vi "LoadController.vi"(8 "error in (no error)":errorcluster, 10 "Actor In":refnum<class "Actor.lvclass">, 11 "Microscope in":refnum<class "Microscope.lvclass">) -> (0 "error out":errorcluster, 3 "Microscope out":refnum<class "Microscope.lvclass">)   [LabVIEW 2020, in "Microscope.lvlib" / "Microscope.lvclass"]
uses:
  Microscope.lvclass
  <vilib>/ActorFramework/Actor/Actor.lvclass
  Component/Device/Device/DataExchange.ctl
  ViewController/Microscope Controller/MicroscopeController.lvclass
  C:/Program Files/National Instruments/LabVIEW 2020/vi.lib/ActorFramework/Actor/Actor.lvclass
  Microscope.lvclass/Microscope.ctl
  Interface/DataListener Messages/OnDataChange Msg/OnDataChange Msg.lvclass/OnDataChange Msg.ctl
  <vilib>/ActorFramework/Message Enqueuer/Message Enqueuer.lvclass/Message Enqueuer.ctl
  <vilib>/ActorFramework/Message Enqueuer/Enqueue.vi
  Interface/DataListener Messages/OnDataChange Msg/OnDataChange Msg.lvclass
  C:/Program Files/National Instruments/LabVIEW 2020/vi.lib/ActorFramework/Message/Message.lvclass
  <vilib>/ActorFramework/Message Priority Queue/Priority Enqueue.vi
  Component/Device/Device/Device.lvclass
  Interface/DataListener/DataListener.lvclass
panel:
  in  "cluster":T1
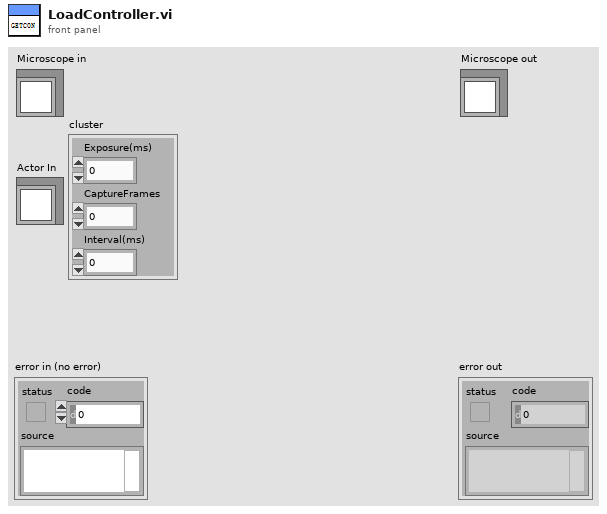
[diagram p1: front panel]
types:
  T1 = cluster{"Exposure(ms)":dbl, "CaptureFrames":dbl, "Interval(ms)":dbl}
  T2 = typedef "DataListener.lvclass/DataExchange.ctl" = cluster{"Source":string, "Destination":string, "Description":string, "value":variant}
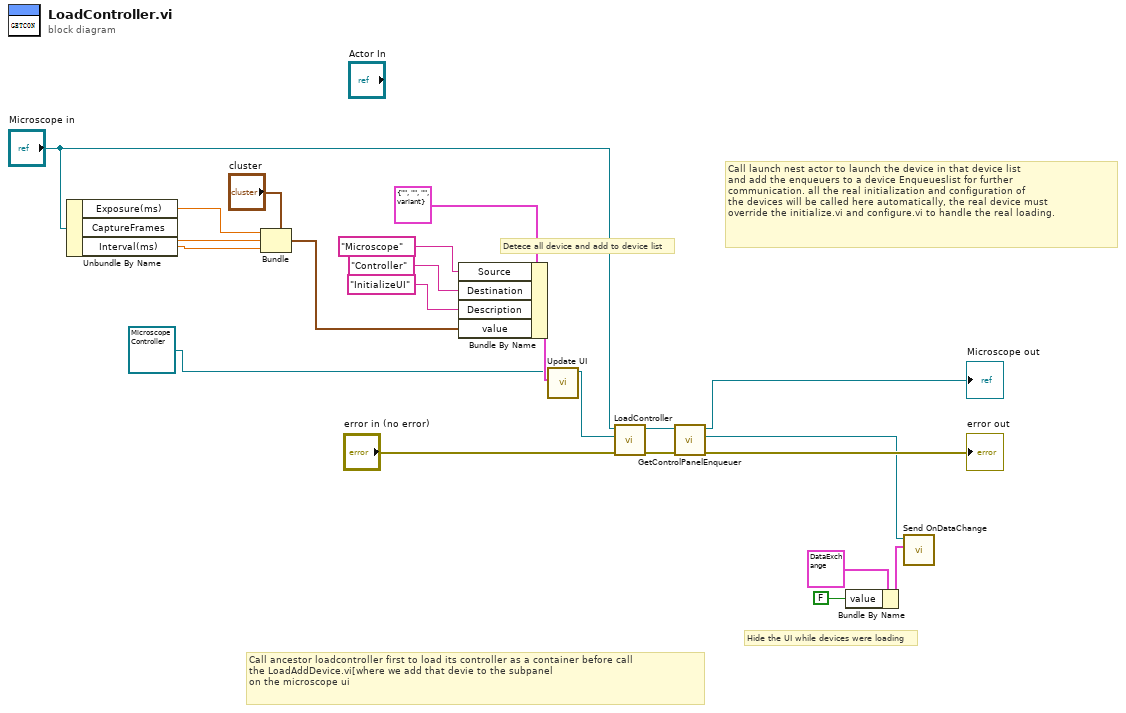
[diagram p0: block diagram]
diagram:
  # "Hide the UI while devices were loading"
  # "Call ancestor loadcontroller first to load its controller as a container before call\nthe LoadAddDevice.vi[where we add that devie to the subpanel \non the microscope ui"
  # "Detece all device and add to device list"
  # "Call launch nest actor to launch the device in that device list\nand add the enqueuers to a device Enqueueslist for further \ncommunication. all the real initialization and configuration of\nthe devices will be called here automatically, the real device must\noverride the initialize.vi and configure.vi to handle the real loading."
  n1 = Unbundle By Name("Microscope in") -> ("Exposure(ms)"=w7:dbl, "CaptureFrames"=w6:dbl, "Interval(ms)"=w5:dbl)
  n2 = Bundle(cluster="cluster", "Exposure(ms)"=w7, "CaptureFrames"=w6, "Interval(ms)"=w5) -> (w3:T1)
  n3 = Bundle By Name(cluster=T2 {"Source"="", "Destination"="", "Description"="", "value"=variant} ("DataExchange"), "Source"="Microscope", "Destination"="Controller", "Description"="InitializeUI", "value"=w3) -> (w12:T2)
  n4 = call "Update UI.vi"("DataExchange"=w12, "Microscope Controller in"=refnum<class "MicroscopeController.lvclass"> refnum ("MicroscopeController.lvlib:MicroscopeController.lvclass")) -> ("Microscope Controller out"=w14:refnum<class "MicroscopeController.lvclass">)  [unwired: 8 in, 1 out]
  n5 = call-parent "LoadController.vi"("error in (no error)"="error in (no error)", "Actor In"=w14, "Device in"="Microscope in") -> ("error out"=w21:errorcluster, "Device out"=w19:refnum<class "Microscope.lvclass">)  [unwired: 7 in]
  n6 = call-dynamic "GetControlPanelEnqueuer.vi"("error in (no error)"=w21, "GRMActor in"=w19) -> ("error out"=→"error out":errorcluster, "ControlViewEnqueuer"=w1:refnum<class "Message Enqueuer.lvclass">, "GRMActor out"=→"Microscope out":refnum<class "Microscope.lvclass">)  [unwired: 7 in]
  n7 = Bundle By Name(cluster=T2 {"Source"="Microscope", "Destination"="Bool", "Description"="ShowUI", "value"=variant} ("DataExchange"), "value"=FALSE) -> (w16:T2)
  n8 = call "Send OnDataChange.vi"("DataExchange"=w16, "Message Enqueuer"=w1) -> ()  [unwired: 8 in, 2 out]
